vi "RSZVB Get Discrete Marker.vi"(8 "error in (no error)":errorcluster {"code" format="%.0x"}, 9 "Marker (1)":i32=1, 10 "Channel (Trace) (1)":i32=1, 11 "VISA session":refnum<visa-resource-name>) -> (0 "error out":errorcluster {"code" format="%.0x"}, 2 "Discrete Mode":i32, 3 "dup VISA session":refnum<visa-resource-name>)   [LabVIEW 2011]
doc: "This VI returns if marker no. <Mk> is set to continuous or discrete mode.\n\nRemote-control command(s):\nCALCulate<Ch/Tr>:MARKer<Mk>:MODE?"
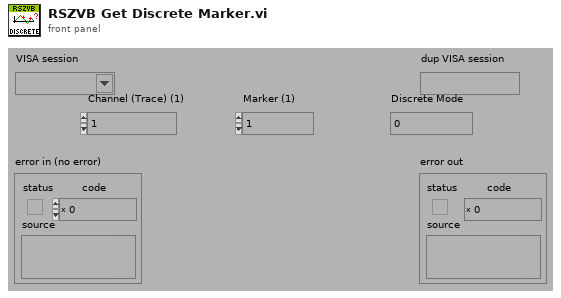
[diagram p1: front panel]
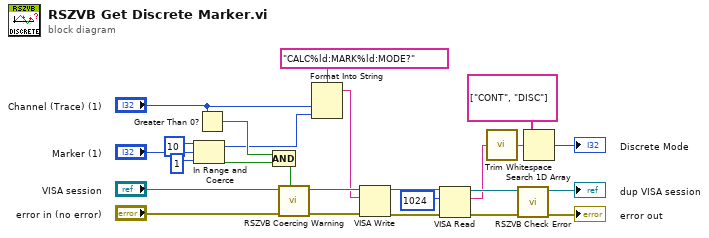
[diagram p0: block diagram]
diagram:
  n1 = In Range and Coerce(upper limit=10, x="Marker (1)", lower limit=1) -> (coerced(x)=w16:i32, In Range?=w17:bool)
  n2 = Greater Than 0?(x="Channel (Trace) (1)") -> (x > 0?=w20:bool)
  n3 = Compound Arithmetic op=AND(w20, w17) -> (w22:bool)
  n4 = call "RSZVB Coercing Warning.vi"("In Range?"=w22, "error in (no error)"="error in (no error)", "VISA session"="VISA session") -> ("error out"=w23:errorcluster, "dup VISA session"=w24:refnum<visa-resource-name>)  [unwired: 7 in]
  n5 = Format Into String(format string="CALC%ld:MARK%ld:MODE?", "Channel (Trace) (1)", w16) -> (resulting string=w21:string)  [unwired: 2 in, 1 out]
  n6 = VISA Write(VISA resource name=w24, write buffer=w21, error in (no error)=w23) -> (VISA resource name out=w5:refnum<visa-resource-name>, error out=w6:errorcluster)  [unwired: 1 out]
  n7 = VISA Read(VISA resource name=w5, byte count=u32 1024 ("byte count (0)"), error in (no error)=w6) -> (VISA resource name out=w10:refnum<visa-resource-name>, read buffer=w2:string, error out=w9:errorcluster)  [unwired: 1 out]
  n8 = call <vilib>:"Trim Whitespace.vi"("string"=w2) -> ("trimmed string"=w1:string)  [unwired: 1 in]
  n9 = call "RSZVB Check Error.vi"("error in (no error)"=w9, "VISA session"=w10) -> ("error out"=→"error out":errorcluster, "dup VISA session"=→"dup VISA session":refnum<visa-resource-name>)  [unwired: 8 in]
  n10 = Search 1D Array(1D array=string[] ["CONT", "DISC"] ("array 2"), element=w1) -> (index of element=→"Discrete Mode":i32)  [unwired: 1 in]
